vi "Write Load Cell Excitation.vi"(10 "Load Cell Excitation":dbl[unit] format="%.1f", 11 "ForceSensorCalculator in":refnum<class "ForceSensorCalculator.lvclass">) -> (3 "ForceSensorCalculator out":refnum<class "ForceSensorCalculator.lvclass">)   [LabVIEW 2015, in "ForceSensorCalculator.lvlib" / "ForceSensorCalculator.lvclass"]
uses:
  <userlib>/Common/Devices/ForceSensorCalculator/ForceSensorCalculator/ForceSensorCalculator.lvclass
  <userlib>/Common/Devices/ForceSensorCalculator/ForceSensorCalculator/ForceSensorCalculator.lvclass/ForceSensorCalculator.ctl
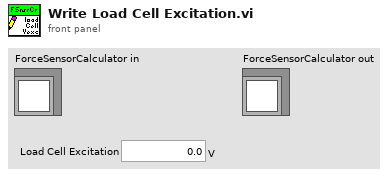
[diagram p1: front panel]
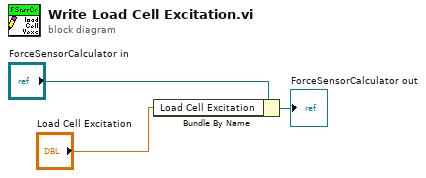
[diagram p0: block diagram]
diagram:
  n1 = Bundle By Name(cluster="ForceSensorCalculator in", "Load Cell Excitation"="Load Cell Excitation") -> (→"ForceSensorCalculator out":refnum<class "ForceSensorCalculator.lvclass">)
